vi "UpdatePublishers.vi"(2 "PubSub":T2, 3 "ROS_Master in":T1) -> (1 "ROS_Master out":T1)   [LabVIEW 2016]
doc: "Updates ROS master with publishers"
uses:
  ROS_Master/ROS_Master.ctl
  ROS_Master/ROS_Topic.ctl
  ROS_Master/ROS_Node.ctl
  ROS_Master/ROS_Service.ctl
panel:
  out "reply XML":string[](array[string])
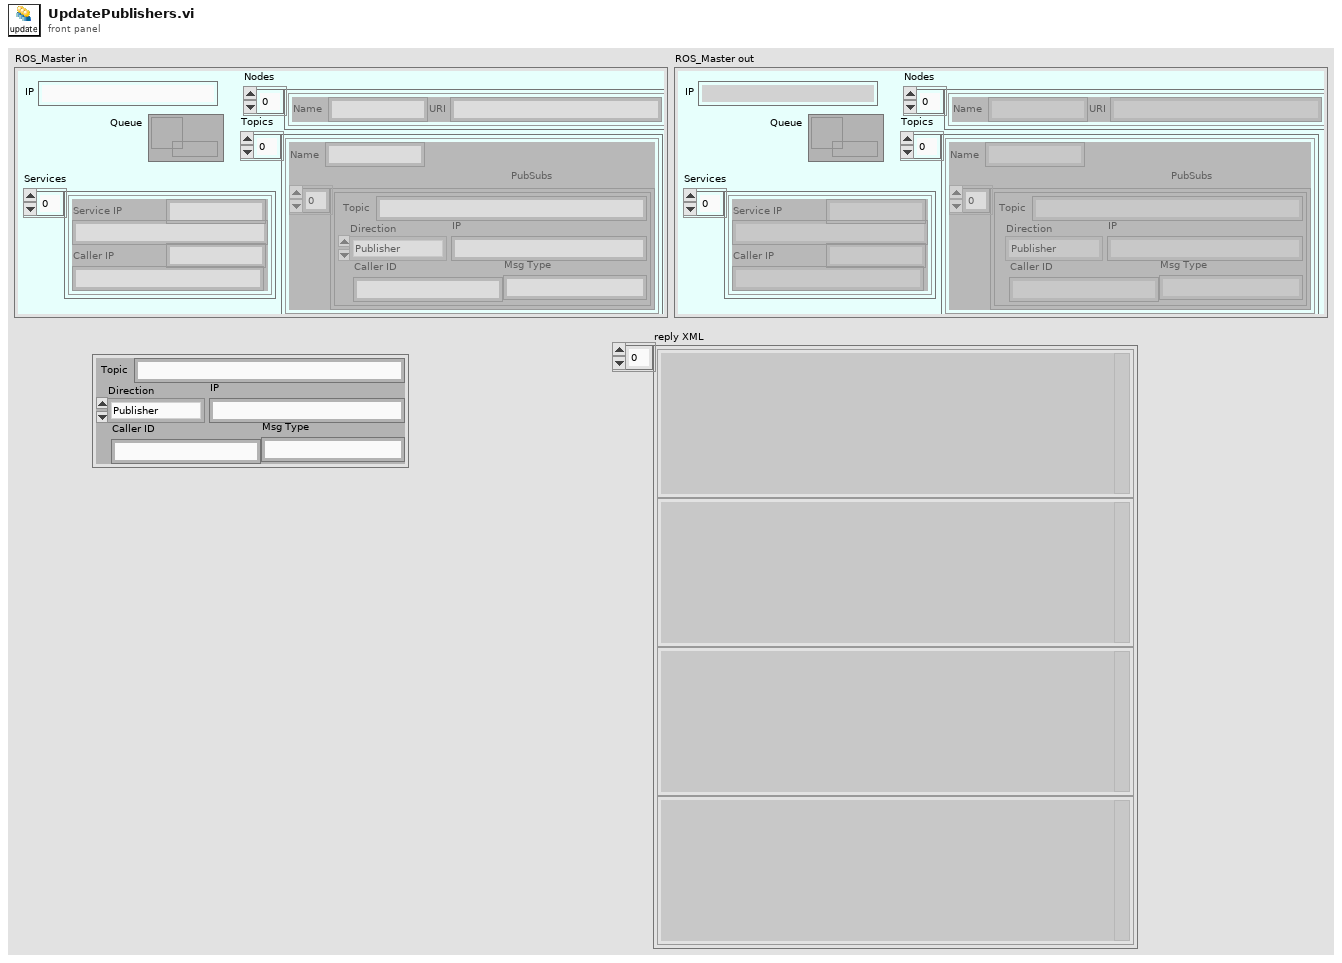
[diagram p1: front panel]
types:
  T1 = typedef "ROS_Master.ctl" = cluster{"IP":string, "Topics":cluster{"Name":string, "PubSubs":T2[]}[], "Nodes":T3[], "Services":T4[], "Queue":refnum<queue>}
  T2 = typedef "ROS_Topic.ctl" = cluster{"Caller ID":string, "IP":string, "Msg Type":string, "Direction":enum16{"Publisher", "Subscriber"}, "Topic":string}
  T3 = typedef "ROS_Node.ctl" = cluster{"Name":string, "URI":string}
  T4 = typedef "ROS_Service.ctl" = cluster{"Service":string, "Service IP":string, "Caller IP":string, "Caller ID":string}
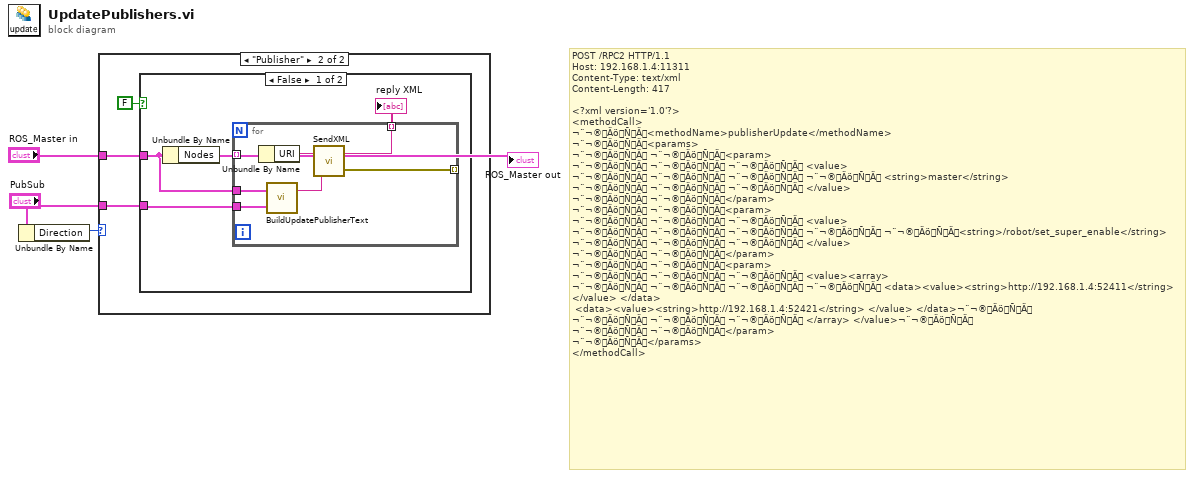
[diagram p0: block diagram]
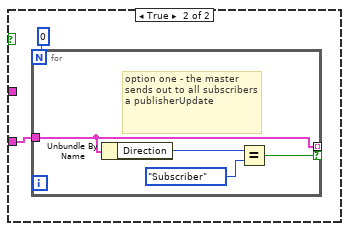
[diagram p3: hidden frame]
diagram:
  # "POST /RPC2 HTTP/1.1\nHost: 192.168.1.4:11311\nContent-Type: text/xml\nContent-Length: 417\n\n<?xml version='1.0'?>\n<methodCall>\n¬¨¬®ÄöÑÄ<methodName>publisherUpdate</methodName>\n¬¨¬®ÄöÑÄ<params>\n¬¨¬®ÄöÑÄ ¬¨¬®ÄöÑÄ<param>\n¬¨¬®ÄöÑÄ ¬¨¬®ÄöÑÄ ¬¨¬®ÄöÑÄ <value>\n¬¨¬®ÄöÑÄ ¬¨¬®ÄöÑÄ ¬¨¬®ÄöÑÄ ¬¨¬®ÄöÑÄ <string>master</string>\n¬¨¬®ÄöÑÄ ¬¨¬®ÄöÑÄ ¬¨¬®ÄöÑÄ </value>\n¬¨¬®ÄöÑÄ ¬¨¬®ÄöÑÄ</param>\n¬¨¬®ÄöÑÄ ¬¨¬®ÄöÑÄ<param>\n¬¨¬®ÄöÑÄ ¬¨¬®ÄöÑÄ ¬¨¬®ÄöÑÄ <value>\n¬¨¬®ÄöÑÄ ¬¨¬®ÄöÑÄ ¬¨¬®ÄöÑÄ ¬¨¬®ÄöÑÄ ¬¨¬®ÄöÑÄ<string>/robot/set_super_enable</string>\n¬¨¬®ÄöÑÄ ¬¨¬®ÄöÑÄ ¬¨¬®ÄöÑÄ </value>\n¬¨¬®ÄöÑÄ ¬¨¬®ÄöÑÄ</param>\n¬¨¬®ÄöÑÄ ¬¨¬®ÄöÑÄ<param>\n¬¨¬®ÄöÑÄ ¬¨¬®ÄöÑÄ ¬¨¬®ÄöÑÄ <value><array>\n¬¨¬®ÄöÑÄ..."
  n1 = Unbundle By Name("PubSub") -> ("Direction"=w2:enum16{"Publisher", "Subscriber"})
  n2 = case shown="\"Publisher\"" w2 {
    tunnel: "PubSub" -> [_ w6]
    tunnel: "ROS_Master in" -> [_ w4]
    frame Default {
    }
    frame "Publisher" {
      n3 = case shown="False" FALSE {
        tunnel: w6 -> [w8 w19]
        tunnel: w4 -> [w9 _]
        frame False {
          n4 = Unbundle By Name(w9) -> ("Nodes"=w10:T3[])
          n5 = for {
            tunnel: w10 -> [w17] mode=indexing
            tunnel: w9 -> [w15]
            tunnel: w8 -> [w14]
            tunnel: [w12] -> w7 mode=indexing
            tunnel: [w11] -> _ mode=indexing
            n6 = Unbundle By Name(w17) -> ("URI"=w16:string)
            n7 = call "BuildUpdatePublisherText.vi"("New Publisher"=w14, "ROS_Master in"=w15) -> ("XML"=w13:string)  [unwired: 1 in]
            n8 = call "SendXML.vi"("Send"=w13, "URI in"=w16) -> ("error out"=w11:errorcluster, "Reply"=w12:string)
          }
          "reply XML" <- w7
        }
        frame True {
          n9 = for {
            N: 0 -> [_]
            tunnel: w19 -> [w21]
            tunnel: [w21] -> _ mode=indexing if=w20
            # "option one - the master sends out to all subscribers\na publisherUpdate"
            n10 = Unbundle By Name(w21) -> ("Direction"=w22:enum16{"Publisher", "Subscriber"})
            n11 = Equal?(x=w22, y=enum16{"Publisher", "Subscriber"}."Subscriber") -> (x = y?=w20:bool)
          }
        }
      }
    }
  }
  "ROS_Master out" <- "ROS_Master in"
